vi "Initialize.vi"(8 "error in (no error)":errorcluster, 10 "DG Nr":i32, 11 "BME_DG_G05 in":refnum<class "BME_DG_G05P2.lvclass">) -> (0 "error out":errorcluster, 3 "BME_DG_G05 out":refnum<class "BME_DG_G05P2.lvclass">)   [LabVIEW 2009, in "BME_DG_G05P2.lvclass"]
uses:
  BME_DG_G05P2.lvclass
  BME_DG_G05P2_Chnl/BME_DG_G05P2_Chnl.lvclass
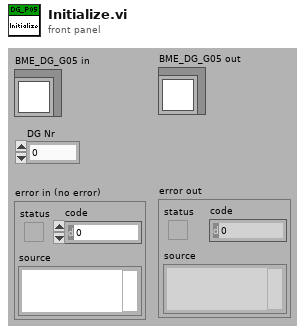
[diagram p1: front panel]
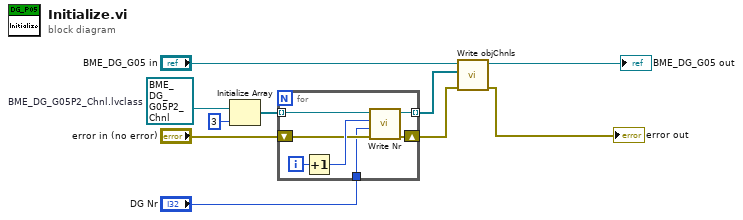
[diagram p0: block diagram]
diagram:
  w1 = refnum<class "BME_DG_G05P2_Chnl.lvclass"> refnum  # BME_DG_G05P2_Chnl.lvclass
  n1 = Initialize Array(w1, 3 ("dimension size")) -> (w7:refnum<class "BME_DG_G05P2_Chnl.lvclass">[])
  n2 = for {
    tunnel: w7 -> [w17] mode=indexing
    tunnel: [w16] -> w6 mode=indexing
    shift-right: [w12] -> w4
    shift-left: "error in (no error)" -> [w13]
    tunnel: "DG Nr" -> [w11]
    i -> [w15]
    n3 = Increment(x=w15) -> (x+1=w14:i32)
    n4 = call-dynamic "Write Nr.vi"("error in (no error)"=w13, "DG Nr"=w11, "Nr"=w14, "BME_DG_Chnl in"=w17) -> ("error out"=w12:errorcluster, "BME_DG_Chnl out"=w16:refnum<class "BME_DG_G05P2_Chnl.lvclass">)  [unwired: 6 in]
  }
  n5 = call-dynamic "Write objChnls.vi"("error in (no error)"=w4, "objChnls"=w6, "BME_DG_Base in"="BME_DG_G05 in") -> ("error out"=→"error out":errorcluster, "BME_DG_Base out"=→"BME_DG_G05 out":refnum<class "BME_DG_G05P2.lvclass">)  [unwired: 7 in]
